vi "inittr.vi"(8 "OptsVer":string="default", 10 "Write/Read":u16(ring) items=["Write", "Read"], 11 "CtlRefs":refnum<vi>[](array[refnum])) -> ()   [LabVIEW 2014]
uses:
  <vilib>/Utility/config.llb/Read Key (Double).vi
  <vilib>/Utility/config.llb/Write Key (Double).vi
  <vilib>/Utility/config.llb/NI_LVConfig.lvlib
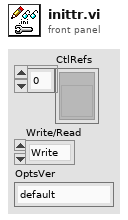
[diagram p1: front panel]
types:
  T1 = typedef "NI_LVConfig.lvlib/Config Data RefNum.ctl" = refnum<k1>
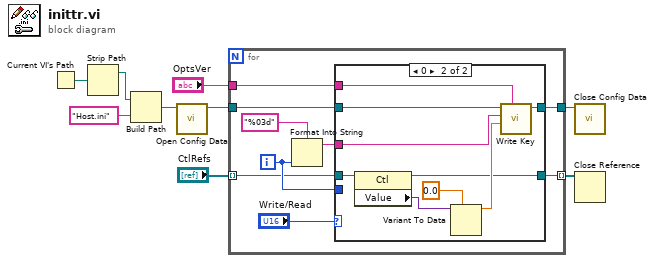
[diagram p0: block diagram]
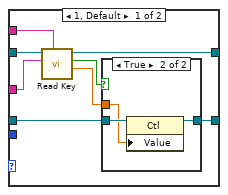
[diagram p2: hidden frame]
diagram:
  n1 = Current VI's Path() -> (path=w9:path)
  n2 = Strip Path(path=w9) -> (stripped path=w8:path)  [unwired: 1 out]
  n3 = Build Path(base path=w8, name or relative path="Host.ini") -> (appended path=w6:path)
  n4 = call <vilib>:"Open Config Data.vi"("configuration file path"=w6) -> ("refnum"=w2:T1)  [unwired: 8 in, 2 out]
  n5 = for {
    tunnel: w2 -> [w18]
    tunnel: "CtlRefs" -> [w11] mode=indexing
    tunnel: [w17] -> w3
    tunnel: "OptsVer" -> [w16]
    tunnel: [w10] -> w1 mode=indexing
    i -> [w12]
    n6 = Format Into String(format string="%03d", w12) -> (resulting string=w13:string)  [unwired: 2 in, 1 out]
    n7 = case shown="0" "Write/Read" {
      tunnel: w18 -> [w26 w39]
      tunnel: [w25 w38] -> w17
      tunnel: w16 -> [w24 w37]
      tunnel: w13 -> [w21 w34]
      tunnel: w12 -> [_ _]
      tunnel: w11 -> [w20 w33]
      tunnel: [w19 w31] -> w10
      frame 1, Default {
        n8 = call-poly <vilib>:"Read Key.vi"("section"=w24, "key"=w21, "refnum"=w26) -> ("value"=w22:dbl, "found?"=w23:bool, "refnum out"=w25:T1)  [unwired: 5 in, 1 out]
        n9 = case shown="True" w23 {
          tunnel: w22 -> [_ w29]
          tunnel: w20 -> [w27 w30]
          tunnel: [w27 w28] -> w19
          frame False {
          }
          frame True {
            n10 = property class="Ctl"(reference=w30, "Value"=w29) -> (reference out=w28:refnum<vi>)  [unwired: 1 in, 1 out]
          }
        }
      }
      frame 0 {
        n11 = property class="Ctl"(reference=w33) -> (reference out=w31:refnum<vi>, "Value"=w32:variant)  [unwired: 1 in, 1 out]
        n12 = Variant To Data(type=0.0, Variant=w32) -> (data=w35:dbl)  [unwired: 1 in, 1 out]
        n13 = call-poly <vilib>:"Write Key.vi"("section"=w37, "value"=w35, "key"=w34, "refnum"=w39) -> ("refnum out"=w38:T1)  [unwired: 5 in, 2 out]
      }
    }
  }
  n14 = call <vilib>:"Close Config Data.vi"("refnum"=w3) -> ()  [unwired: 9 in, 2 out]
  n15 = Close Reference(reference=w1) -> ()  [unwired: 1 in, 1 out]
